vi "ASS1-3SIN.vi"() -> ()   [LabVIEW 2018]
uses:
  Control 2.ctl
  Control 1.ctl
  <vilib>/measure/NI_MABase.lvlib
panel:
  in  "frequency":dbl=10.0 format="%0.2p"
  out "SIN WAVE 2":dynamicdata(graph)
  out "SIN WAVE 3":dynamicdata(graph)
  out "SIN WAVE1":dynamicdata(graph)
  out "3 SIN WAVES":waveform(dbl)(graph)
  in  "amplitude 3":dbl=1.0 format="%0.2p"
  in  "amplitude 2":dbl=1.0 format="%0.2p"
  in  "amplitude":dbl=1.0 format="%0.2p"
  in  "frequency 3":T1=10.0 format="%0.2p"
  in  "frequency 2":T2=10.0 format="%0.2p"
  in  "sampling info":cluster{"Fs":dbl, "#s":dbl}={"Fs"=1000.0, "#s"=1000.0} {"Fs" format="%.2p"}
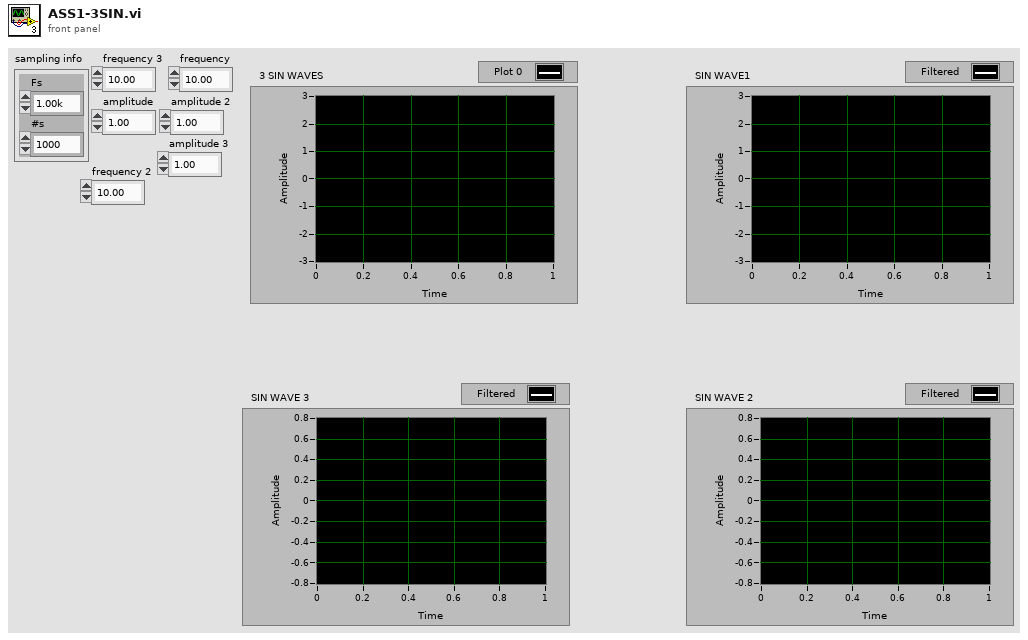
[diagram p1: front panel]
types:
  T1 = typedef "Control 1.ctl" = dbl
  T2 = typedef "Control 2.ctl" = dbl
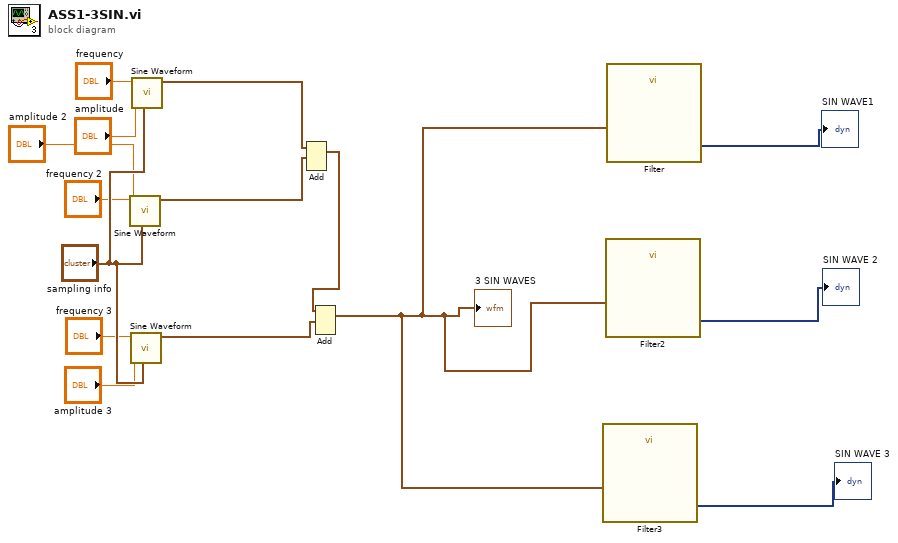
[diagram p0: block diagram]
diagram:
  n1 = call <vilib>:"Sine Waveform.vi"("sampling info"="sampling info", "amplitude"="amplitude 2", "frequency"="frequency 2") -> ("signal out"=w14:waveform(dbl))  [unwired: 7 in, 1 out]
  n2 = call <vilib>:"Sine Waveform.vi"("sampling info"="sampling info", "amplitude"="amplitude 3", "frequency"="frequency 3") -> ("signal out"=w12:waveform(dbl))  [unwired: 7 in, 1 out]
  n3 = call <vilib>:"Sine Waveform.vi"("sampling info"="sampling info", "amplitude"="amplitude", "frequency"="frequency") -> ("signal out"=w15:waveform(dbl))  [unwired: 7 in, 1 out]
  n4 = Add(1:w14, 2:w15) -> (0:w13:waveform(dbl))  [unwired: 1 in, 1 out]
  n5 = Add(1:w12, 2:w13) -> (0:w2:waveform(dbl))  [unwired: 1 in, 1 out]
  "3 SIN WAVES" <- w2
  n6 = call "Filter3"("Signal"=w2) -> ("Filtered Signal"=→"SIN WAVE 3":dynamicdata)  [unwired: 9 in, 1 out]
  n7 = call "Filter2"("Signal"=w2) -> ("Filtered Signal"=→"SIN WAVE 2":dynamicdata)  [unwired: 9 in, 1 out]
  n8 = call "Filter"("Signal"=w2) -> ("Filtered Signal"=→"SIN WAVE1":dynamicdata)  [unwired: 9 in, 1 out]
